vi "Wait Progress Bar.vi"(8 "error in (no error)":errorcluster, 9 "Message [Shutting Down...]":string="Shutting Down...", 10 "wait (ms)":u32=1000) -> (0 "error out":errorcluster)   [LabVIEW 2019, in "instrument.PPMS.lvclass"]
uses:
  instrument.PPMS.lvclass
panel:
  out "Message":string="Shutting Down..."
  out "Slide":i32(slide) scale=0.0..100.0
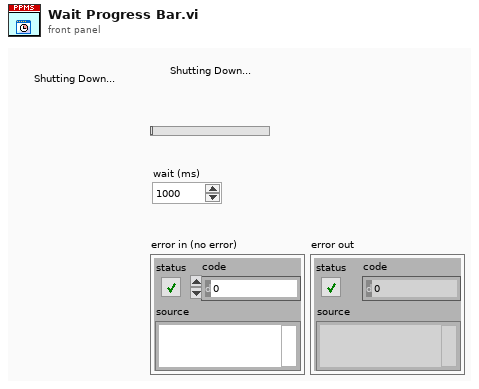
[diagram p1: front panel]
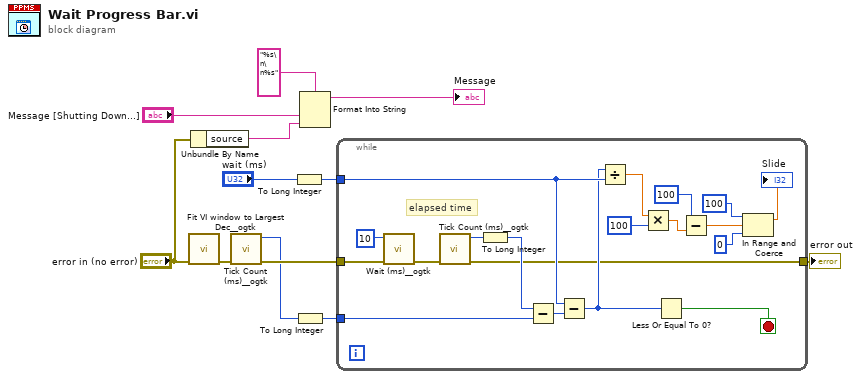
[diagram p0: block diagram]
diagram:
  n1 = call <userlib>:"Fit VI window to Largest Dec__ogtk.vi"("error in (no error)"="error in (no error)") -> ("error out"=w7:errorcluster)  [unwired: 5 in, 1 out]
  n2 = Unbundle By Name("error in (no error)") -> ("source"=w2:string)
  n3 = call <userlib>:"Tick Count (ms)__ogtk.vi"("error in (no error)"=w7) -> ("error out"=w12:errorcluster, "millisecond timer value"=w11:u32)  [unwired: 9 in]
  n4 = To Long Integer(number="wait (ms)") -> (32bit integer=w9:i32)
  n5 = To Long Integer(number=w11) -> (32bit integer=w8:i32)
  n6 = Format Into String(format string="%s\n\n%s", "Message [Shutting Down...]", w2) -> (resulting string=→"Message":string)  [unwired: 2 in, 1 out]
  n7 = while {
    tunnel: w12 -> [w31]
    tunnel: w8 -> [w20]
    tunnel: w9 -> [w22]
    tunnel: [w19] -> w6
    stop <- w28 stop-if-true
    # "elapsed time"
    n8 = call <userlib>:"Wait (ms)__ogtk.vi"("error in (no error)"=w31, "milliseconds to wait"=u32 10) -> ("error out"=w30:errorcluster)  [unwired: 8 in, 1 out]
    n9 = call <userlib>:"Tick Count (ms)__ogtk.vi"("error in (no error)"=w30) -> ("error out"=w19:errorcluster, "millisecond timer value"=w26:u32)  [unwired: 9 in]
    n10 = To Long Integer(number=w26) -> (32bit integer=w25:i32)
    n11 = Subtract(x=w25, y=w20) -> (x-y=w24:i32)
    n12 = Subtract(x=w22, y=w24) -> (x-y=w21:i32)
    n13 = Divide(x=w21, y=w22) -> (x/y=w18:dbl)
    n14 = Multiply(x=w18, y=100) -> (x*y=w13:dbl)
    n15 = Less Or Equal To 0?(x=w21) -> (x <= 0?=w28:bool)
    n16 = Subtract(x=100 ("y"), y=w13) -> (x-y=w17:dbl)
    n17 = In Range and Coerce(upper limit=100, x=w17, lower limit=0) -> (coerced(x)=→"Slide":dbl)  [unwired: 1 out]
  }
  "error out" <- w6
